vi "Sub_truncate_buffer.vi"(5 "array":dbl[](array[numeric]), 10 "samples":i32) -> (4 "array":dbl[](array[numeric]))   [LabVIEW 2021]
panel:
  out "size(s)":i32
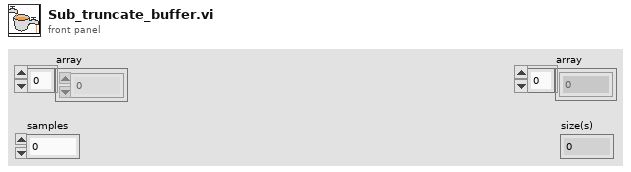
[diagram p1: front panel]
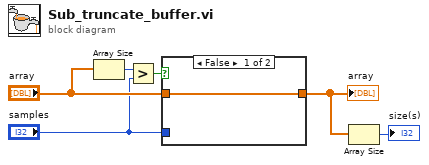
[diagram p0: block diagram]
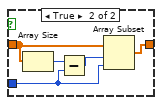
[diagram p2: hidden frame]
diagram:
  n1 = Array Size(array="array") -> (size(s)=w6:i32)
  n2 = Greater?(x=w6, y="samples") -> (0:w5:bool)
  n3 = case shown="False" w5 {
    tunnel: "samples" -> [_ w9]
    tunnel: "array" -> [w7 w12]
    tunnel: [w7 w8] -> w2
    frame False {
    }
    frame True {
      n4 = Array Size(array=w12) -> (size(s)=w11:i32)
      n5 = Subtract(x=w11, y=w9) -> (x-y=w10:i32)
      n6 = Array Subset(array=w12, index=w10, length=w9) -> (w8:dbl[])
    }
  }
  "array" <- w2
  n7 = Array Size(array=w2) -> (size(s)=→"size(s)":i32)
